vi "NameIsWhiteSpace.vi"(11 "User Input":T1) -> (3 "IsWhiteSpaceOrEmpty?":bool)   [LabVIEW 2017]
uses:
  Ctrl/UserInput.ctl
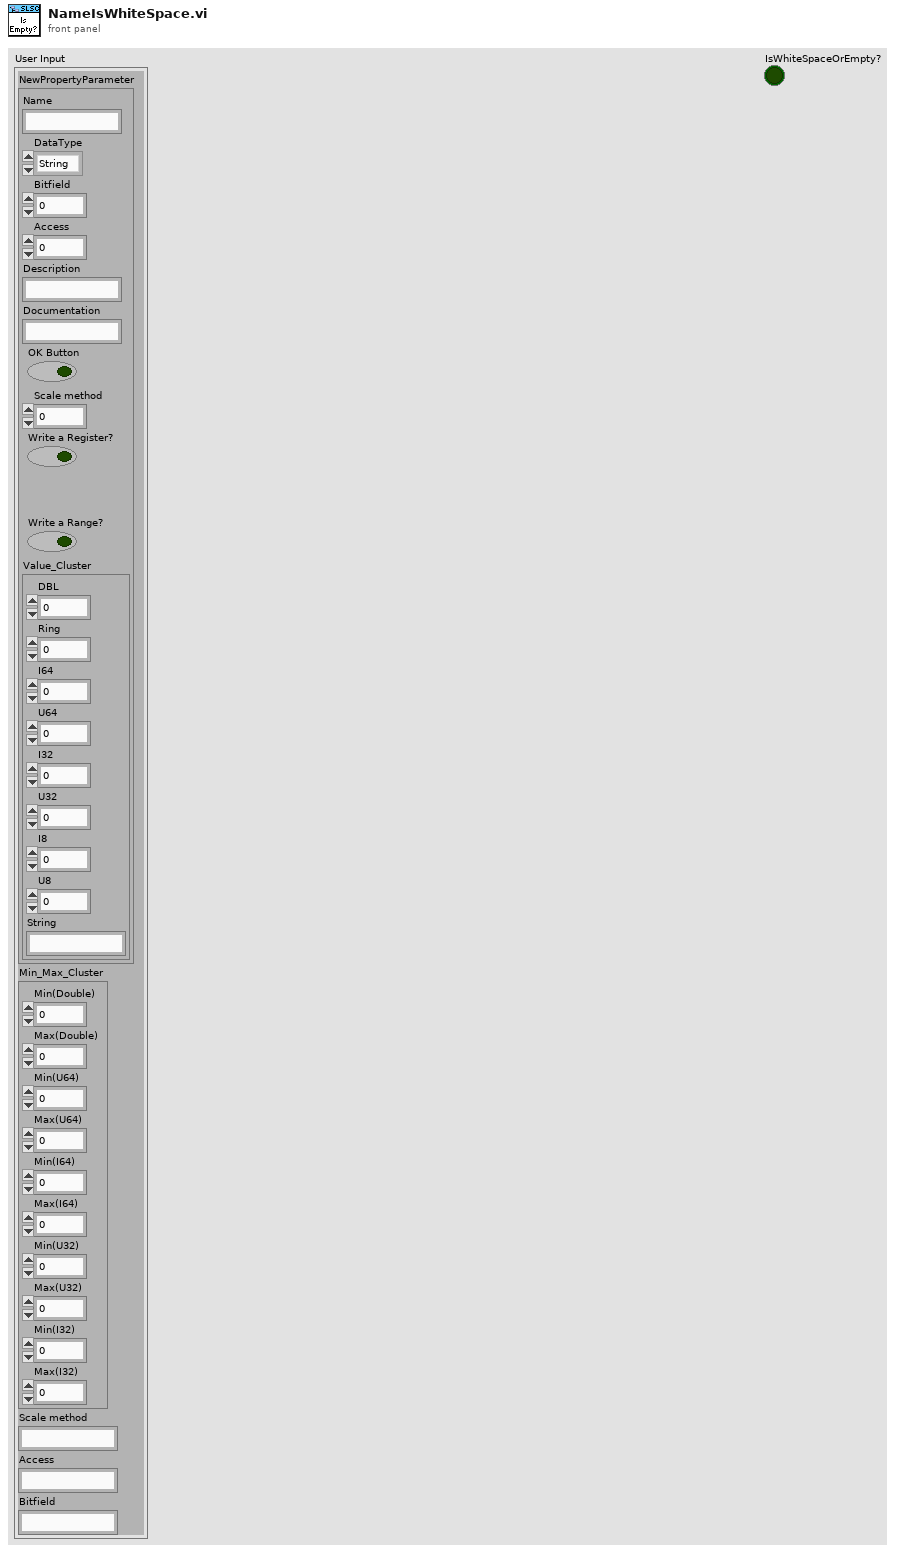
[diagram p1: front panel]
types:
  T1 = typedef "UserInput.ctl" = cluster{"NewPropertyParameter":cluster{"Name":string, "DataType":enum16{"String", "Double", "U64", "I64", "U32", "I32", "Bool"}, "Bitfield":u16, "Access":u16, "Description":string, "Documentation":string, "OK Button":bool, "Scale method":u16, "Write a Register?":bool, "Write a Range?":bool, "Value_Cluster":cluster{"DBL":dbl, "Ring":u16, "I64":i64, "U64":u64, "I32":i32, "U32":u32, "I8":i8, "U8":u8, "String":string}}, "Min_Max_Cluster":cluster{"Min(Double)":dbl, "Max(Double)":dbl, "Min(U64)":u64, "Max(U64)":u64, "Min(I64)":i64, "Max(I64)":i64, "Min(U32)":u32, "Max(U32)":u32, "Min(I32)":i32, "Max(I32)":i32}, "Scale method":string, "Access":string, "Bitfield":string}
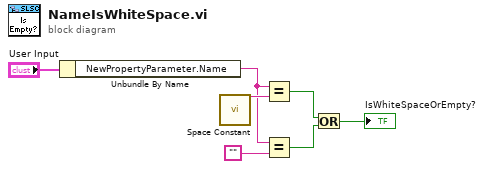
[diagram p0: block diagram]
diagram:
  n1 = Unbundle By Name("User Input") -> ("NewPropertyParameter.Name"=w5:string)
  n2 = call <vilib>:"Space Constant.vi"() -> ("String"=w6:string)
  n3 = Equal?(x=w5, y=w6) -> (x = y?=w3:bool)
  n4 = Equal?(x=w5, y="") -> (x = y?=w2:bool)
  n5 = Or(x=w3, y=w2) -> (x .or. y?=→"IsWhiteSpaceOrEmpty?":bool)
